vi "Periodic Tasks.vi"(8 "error in":errorcluster) -> ()   [LabVIEW 2019]
doc: "This VI runs in parallel to other tasks. It can contain as many user-defined periodic loops as you need. These can carry out PID or other sorts of timed response."
uses:
  <vilib>/Rock Robotics/WPI/Utilities/WPI_GetSetVariantRefNum.vi
  <vilib>/Rock Robotics/Network Tables/NT Read Number.vi
  <vilib>/Rock Robotics/Network Tables/NT Read Boolean.vi
  <vilib>/Rock Robotics/Network Tables/NT Write Number.vi
  Downloads/Global 2.vi
  ultraG.vi
panel:
  out "sensonic":bool
  out "sensonic":bool
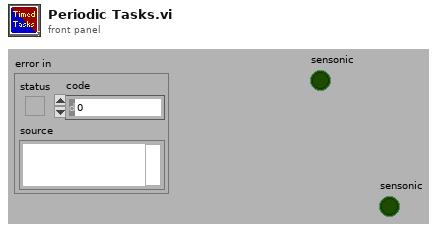
[diagram p1: front panel]
types:
  T1 = typedef "WPI_JoystickDevRef.ctl" = cluster{"Device":T2}
  T2 = typedef "WPI_JoystickDeviceEnum.ctl" = enum16{"USB 0", "USB 1", "USB 2", "USB 3", "USB 4", "USB 5"}
  T3 = typedef "WPI_RobotDriveDevRef.ctl" = cluster{"DevStatus":errorcluster, "Motors[]":T4[], "Square Inputs":bool, "Max Output":dbl}
  T4 = typedef "WPI_MotorControlDeviceRef.ctl" = cluster{"DeviceStatus":errorcluster, "Type":T5, "PWM":cluster{"PWM Channel":T6, "DeadBand":T7}, "CAN":cluster{"Device Number":u8, "SetOutput VI Ref":variant, "GetOutput VI Ref":variant, "Enable VI Ref":variant, "Disable VI Ref":variant, "Data":variant}, "Invert":bool, "DIO PWM":cluster{"PWM \"Enable\" Channel":T6, "DIOChannel":T8, "PWM Rate":dbl}}
  T5 = typedef "WPI_MotorControlType.ctl" = enum16{"PWM", "CAN", "DIO PWM"}
  T6 = typedef "FPGA_DIOPWMChannel.ctl" = enum8{"PWM 0", "PWM 1", "PWM 2", "PWM 3", "PWM 4", "PWM 5", "PWM 6", "PWM 7", "PWM 8", "PWM 9", "PWM MXP 0", "PWM MXP 1", "PWM MXP 2", "PWM MXP 3", "PWM MXP 4", "PWM MXP 5", "PWM MXP 6", "PWM MXP 7", "PWM MXP 8", "PWM MXP 9", "Invalid"}
  T7 = typedef "WPI_PWMDeadband.ctl" = cluster{"Name":string, "maxPositivePwm":i32, "minPositivePwm":i32, "centerPwm":i32, "maxNegativePwm":i32, "minNegativePwm":i32, "angularRange":u16}
  T8 = typedef "FPGA_DIOChannel.ctl" = enum8{"DIO 0", "DIO 1", "DIO 2", "DIO 3", "DIO 4", "DIO 5", "DIO 6", "DIO 7", "DIO 8", "DIO 9", "DIO MXP 0", "DIO MXP 1", "DIO MXP 2", "DIO MXP 3", "DIO MXP 4", "DIO MXP 5", "DIO MXP 6", "DIO MXP 7", "DIO MXP 8", "DIO MXP 9", "DIO MXP 10", "DIO MXP 11", "DIO MXP 12", "DIO MXP 13", "DIO MXP 14", "DIO MXP 15", "SPI Port CS1", "SPI Port CS2", "SPI Port CS3", "SPI Port MISO", "SPI Port MOSI", "Invalid"}
  T9 = cluster{"JoystickDevRef":T1, "RobotDriveDevRef":T3}
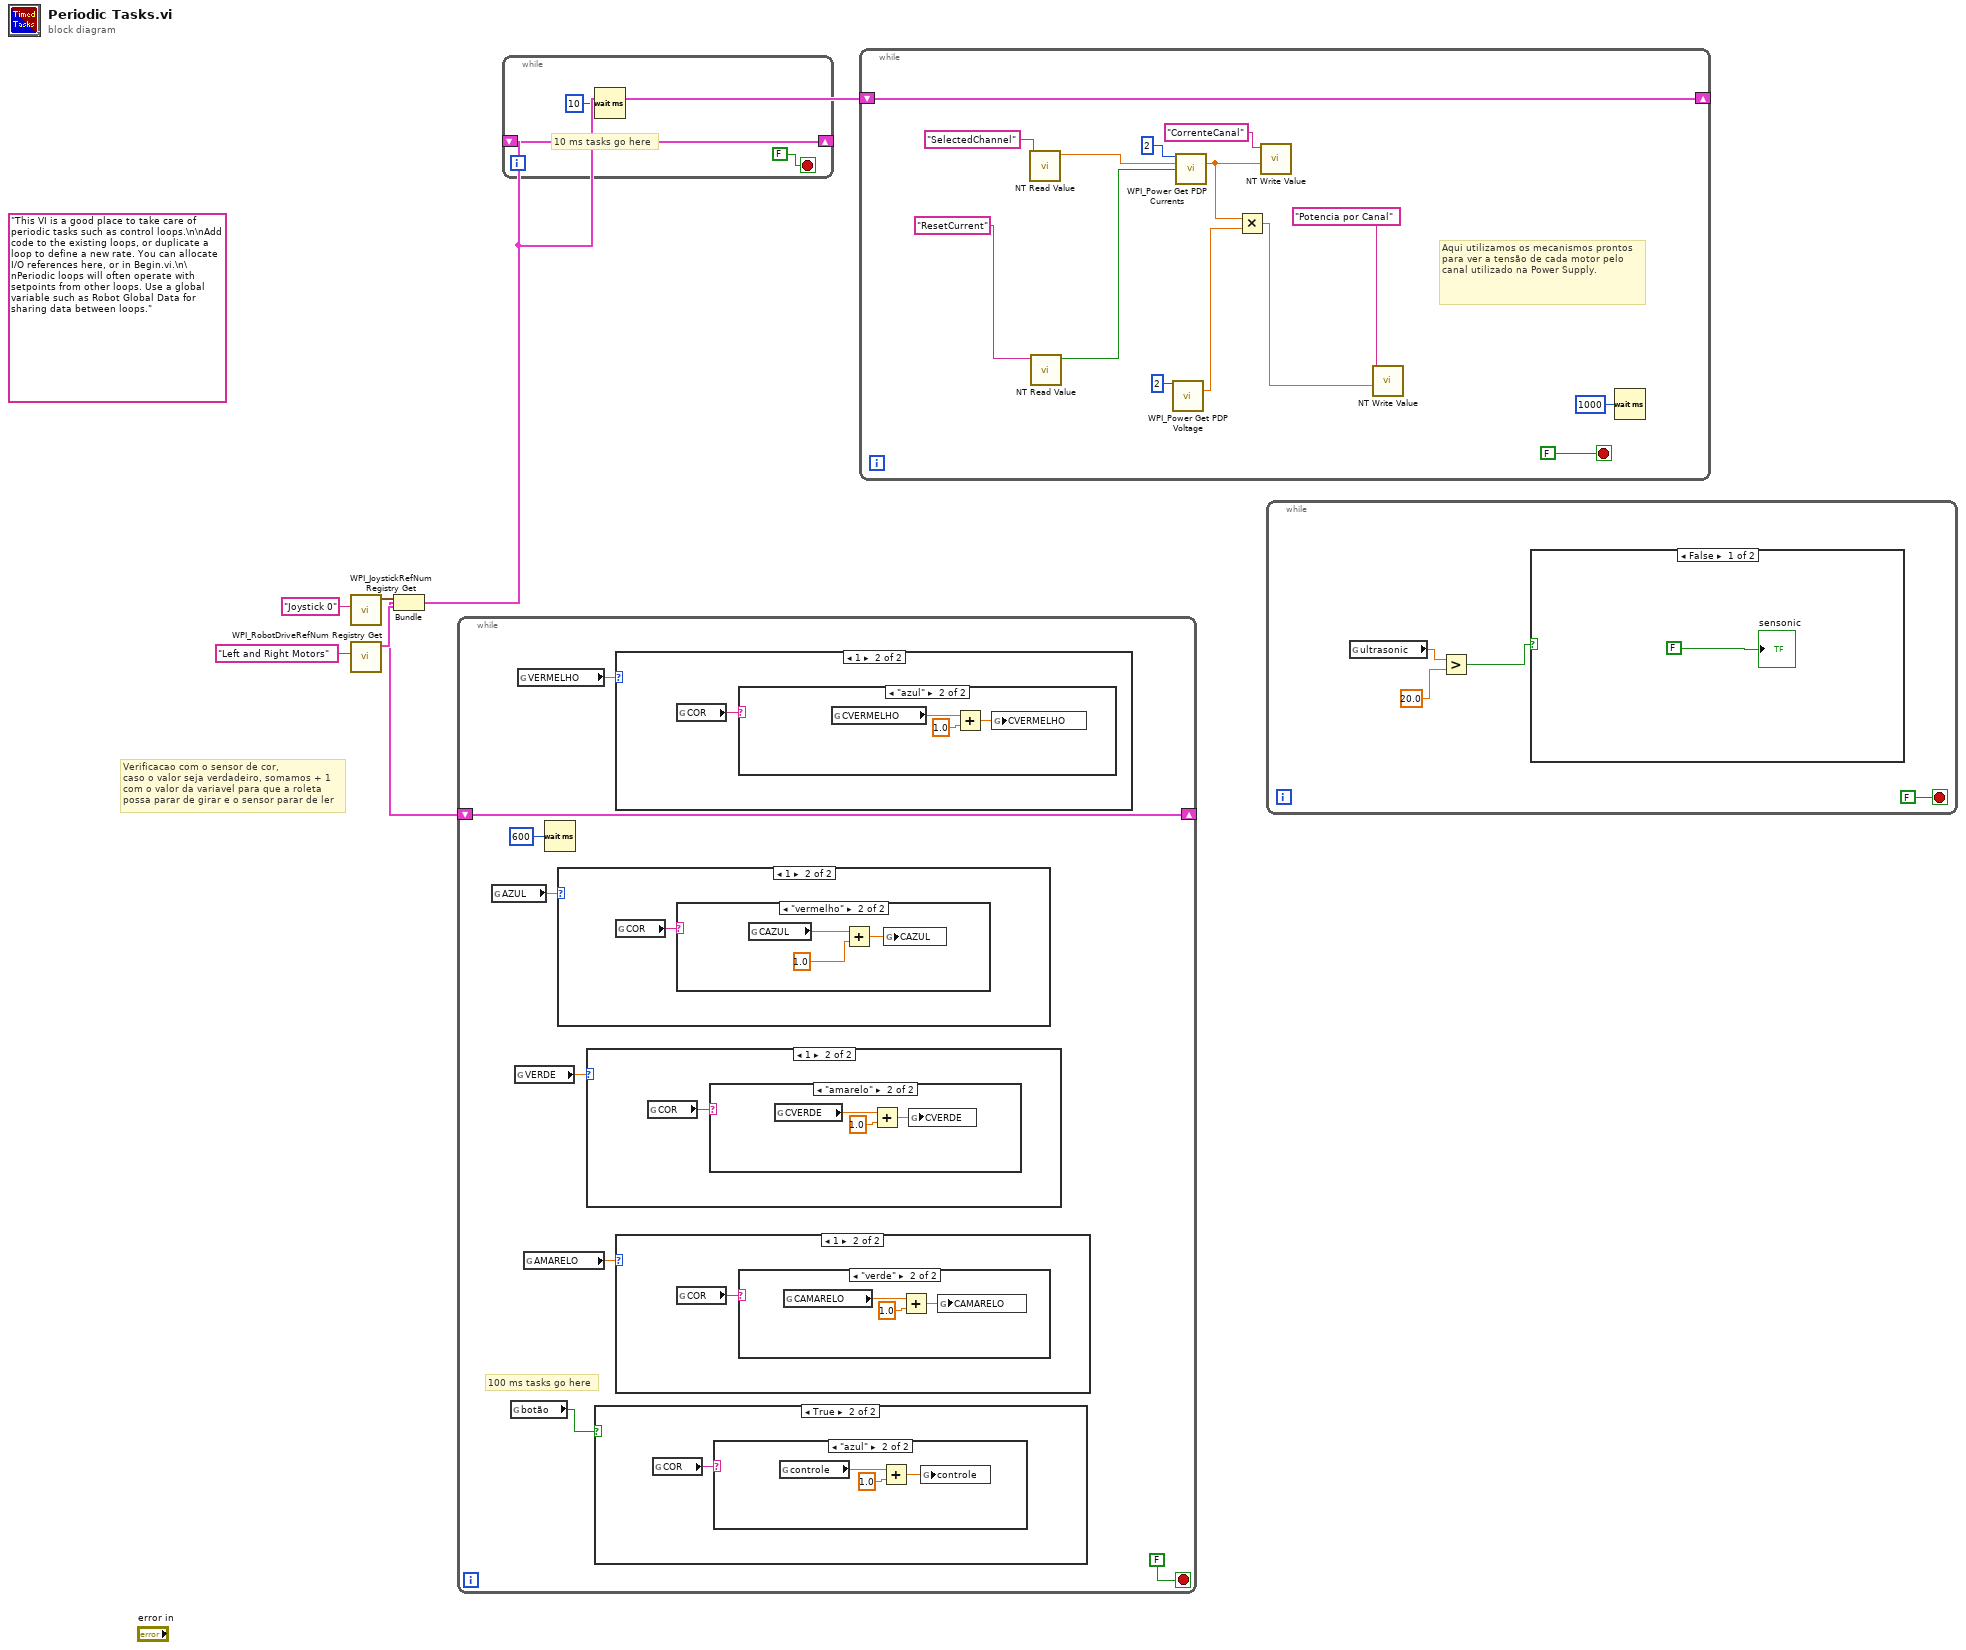
[diagram p0: block diagram]
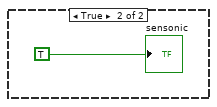
[diagram p2: hidden frame]
diagram:
  (unwired) "This VI is a good place to take care of periodic tasks such as control loops.\n\nAdd code to the existing loops, or duplicate a loop to define a new rate. You can allocate I/O references here, or in Begin.vi.\n\nPeriodic loops will often operate with setpoints from other loops. Use a global variable such as Robot Global Data for sharing data between loops."
  # "Verificacao com o sensor de cor,\ncaso o valor seja verdadeiro, somamos + 1\ncom o valor da variavel para que a roleta \npossa parar de girar e o sensor parar de ler"
  n1 = call <vilib>:"WPI_JoystickRefNum Registry Get.vi"("refnum name"="Joystick 0") -> ("JoystickDevRef"=w3:T1)  [unwired: 1 in, 9 out]
  n2 = call <vilib>:"WPI_RobotDriveRefNum Registry Get.vi"("refnum name"="Left and Right Motors") -> ("RobotDriveDevRef"=w2:T3)  [unwired: 1 in, 9 out]
  n3 = Bundle("JoystickDevRef"=w3, "RobotDriveDevRef"=w2) -> (w1:T9)  [unwired: 1 out]
  n4 = while {
    shift-right: [w11] -> _
    shift-left: w1 -> [w11]
    stop <- FALSE stop-if-true
    # "100 ms tasks go here"
    n5 = global read "Global 2.vi" "AZUL"() -> (w10:dbl)
    n6 = global read "Global 2.vi" "botão"() -> (w6:bool)
    n7 = global read "Global 2.vi" "VERDE"() -> (w8:dbl)
    n8 = global read "Global 2.vi" "VERMELHO"() -> (w7:dbl)
    n9 = global read "Global 2.vi" "AMARELO"() -> (w9:dbl)
    n10 = Wait (ms)(milliseconds to wait=u32 600) -> ()  [unwired: 1 out]
    n11 = case shown="1" w10 {
      frame 0, Default {
      }
      frame 1 {
        n12 = global read "Global 2.vi" "COR"() -> (w30:string)
        n13 = case shown="\"vermelho\"" w30 {
          frame "False", Default {
          }
          frame "vermelho" {
            n14 = global read "Global 2.vi" "CAZUL"() -> (w33:dbl)
            n15 = Add(x=w33, y=1.0) -> (x+y=w32:dbl)
            n16 = global write "Global 2.vi" "CAZUL"(w32) -> ()
          }
        }
      }
    }
    n17 = case shown="1" w8 {
      frame 0, Default {
      }
      frame 1 {
        n18 = global read "Global 2.vi" "COR"() -> (w22:string)
        n19 = case shown="\"amarelo\"" w22 {
          frame "False", Default {
          }
          frame "amarelo" {
            n20 = global read "Global 2.vi" "CVERDE"() -> (w25:dbl)
            n21 = Add(x=w25, y=1.0) -> (x+y=w24:dbl)
            n22 = global write "Global 2.vi" "CVERDE"(w24) -> ()
          }
        }
      }
    }
    n23 = case shown="True" w6 {
      frame False {
      }
      frame True {
        n24 = global read "Global 2.vi" "COR"() -> (w14:string)
        n25 = case shown="\"azul\"" w14 {
          frame "False", Default {
          }
          frame "azul" {
            n26 = global read "Global 2.vi" "controle"() -> (w17:dbl)
            n27 = Add(x=w17, y=1.0) -> (x+y=w16:dbl)
            n28 = global write "Global 2.vi" "controle"(w16) -> ()
          }
        }
      }
    }
    n29 = case shown="1" w7 {
      frame 0, Default {
      }
      frame 1 {
        n30 = global read "Global 2.vi" "COR"() -> (w18:string)
        n31 = case shown="\"azul\"" w18 {
          frame "False", Default {
          }
          frame "azul" {
            n32 = global read "Global 2.vi" "CVERMELHO"() -> (w21:dbl)
            n33 = Add(x=w21, y=1.0) -> (x+y=w20:dbl)
            n34 = global write "Global 2.vi" "CVERMELHO"(w20) -> ()
          }
        }
      }
    }
    n35 = case shown="1" w9 {
      frame 0, Default {
      }
      frame 1 {
        n36 = global read "Global 2.vi" "COR"() -> (w26:string)
        n37 = case shown="\"verde\"" w26 {
          frame "False", Default {
          }
          frame "verde" {
            n38 = global read "Global 2.vi" "CAMARELO"() -> (w29:dbl)
            n39 = Add(x=w29, y=1.0) -> (x+y=w28:dbl)
            n40 = global write "Global 2.vi" "CAMARELO"(w28) -> ()
          }
        }
      }
    }
  }
  n41 = while {
    shift-right: [w34] -> _
    shift-left: w1 -> [w34]
    stop <- FALSE stop-if-true
    # "10 ms tasks go here"
    n42 = Wait (ms)(milliseconds to wait=u32 10) -> ()  [unwired: 1 out]
  }
  n43 = while {
    shift-right: [w50] -> _
    shift-left: w1 -> [w50]
    stop <- FALSE stop-if-true
    # "Aqui utilizamos os mecanismos prontos para ver a tensão de cada motor pelo canal utilizado na Power Supply."
    n44 = call-poly <vilib>:"NT Read Value.vi"("Name"="SelectedChannel") -> ("Numeric"=w46:dbl)  [unwired: 9 in, 1 out]
    n45 = call-poly <vilib>:"NT Read Value.vi"("Name"="ResetCurrent") -> ("Boolean"=w45:bool)  [unwired: 9 in, 1 out]
    n46 = call <vilib>:"WPI_Power Get PDP Voltage.vi"("Power Distribution Panel (0)"=u8 2) -> ("voltage (V)"=w41:dbl)  [unwired: 13 in, 1 out]
    n47 = call <vilib>:"WPI_Power Get PDP Currents.vi"("Power Distribution Panel (0)"=u8 2, "PDP Channel"=w46, "Tare Currents?"=w45) -> ("current (A)"=w42:dbl)  [unwired: 10 in, 2 out]
    n48 = Multiply(x=w42, y=w41) -> (x*y=w40:dbl)
    n49 = call-poly <vilib>:"NT Write Value.vi"("Numeric"=w42, "Name"="CorrenteCanal") -> ()  [unwired: 9 in, 1 out]
    n50 = call-poly <vilib>:"NT Write Value.vi"("Numeric"=w40, "Name"="Potencia por Canal") -> ()  [unwired: 9 in, 1 out]
    n51 = Wait (ms)(milliseconds to wait=u32 1000) -> ()  [unwired: 1 out]
  }
  n52 = while {
    stop <- FALSE stop-if-true
    n53 = global read "ultraG.vi" "ultrasonic"() -> (w52:dbl)
    n54 = Greater?(x=w52, y=20.0) -> (0:w53:bool)
    n55 = case shown="False" w53 {
      frame False {
        "sensonic" <- FALSE ("sensonic")
      }
      frame True {
        "sensonic" <- TRUE ("sensonic")
      }
    }
  }
